vi "InitSnakes.vi"(8 "error in (no error)":errorcluster, 11 "SnakeGame in":refnum<class "SnakeGame.lvclass">) -> (0 "error out":errorcluster, 3 "SnakeGame out":refnum<class "SnakeGame.lvclass">)   [LabVIEW 2019, in "RT_Game.lvlib" / "SnakeGame.lvclass"]
uses:
  SnakeGame.lvclass
  C:/Users/FreshBob/Dropbox/VIs/myRIO_GameConsole/RT/RT_Game/Game/Game.lvclass
  Engine/Coordinate.ctl
  Snake/Direction.ctl
  Snake/Snake.lvclass
  Game/Game.lvclass/Game.ctl
  Snake/Snake.lvclass/Snake.ctl
  SnakeGame.lvclass/SnakeGame.ctl
  Game/Read Singleplayer.vi
  Snake/Write Position (Tiles).vi
  Snake/Write Direction.vi
  Snake/Write ScorePosition.vi
  Snake/Write Color.vi
  Snake/Write Length.vi
  Snake/Write tick_rate.vi
  Snake/Write Dead_.vi
  Engine/Engine.lvclass
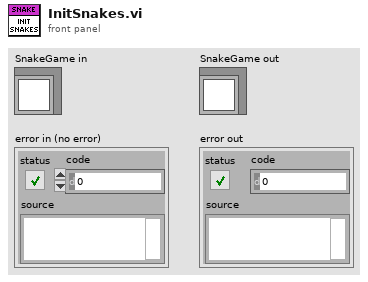
[diagram p1: front panel]
types:
  T1 = typedef "RT_Game.lvlib/Engine.lvclass/Coordinate.ctl" = cluster{"x":dbl, "y":dbl}
  T2 = typedef "RT_Game.lvlib/Snake.lvclass/Direction.ctl" = enum16{"Up", "Left", "Down", "Right"}
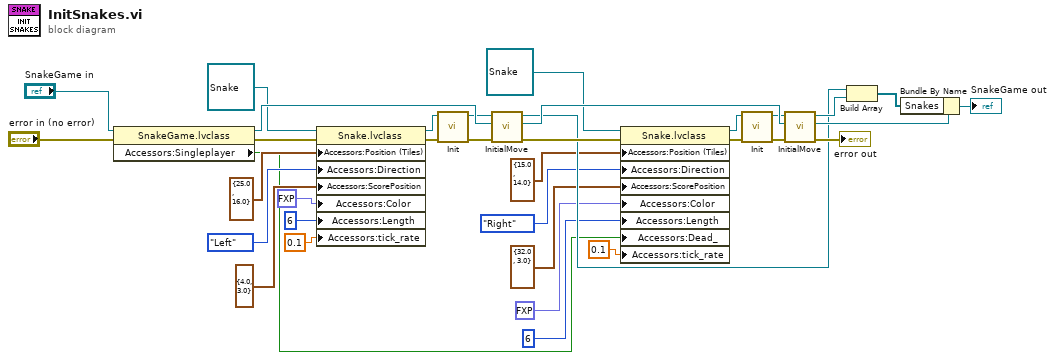
[diagram p0: block diagram]
diagram:
  n1 = property class="SnakeGame.lvclass"(reference="SnakeGame in", error in="error in (no error)") -> (reference out=w35:refnum<class "SnakeGame.lvclass">, error out=w29:errorcluster, "Accessors:Singleplayer"=w1:bool)
  n2 = property class="Snake.lvclass"(reference=refnum<class "Snake.lvclass"> refnum ("RT_Game.lvlib:Snake.lvclass"), error in=w29, "Accessors:Position (Tiles)"=T1 {"x"=25.0, "y"=16.0} ("Position (Tiles)"), "Accessors:Direction"=Direction."Left" ("Direction"), "Accessors:ScorePosition"=T1 {"x"=4.0, "y"=3.0} ("ScorePosition"), "Accessors:Color"=fxp<+,3,3> 1.0 ("Color"), "Accessors:Length"=i16 6 ("Length"), "Accessors:tick_rate"=0.1 ("tick_rate")) -> (reference out=w21:refnum<class "Snake.lvclass">, error out=w20:errorcluster)
  n3 = call-dynamic "Init.vi"("error in (no error)"=w20, "Snake in"=w21) -> ("error out"=w3:errorcluster, "Snake out"=w25:refnum<class "Snake.lvclass">)  [unwired: 8 in]
  n4 = call "InitialMove.vi"("error in (no error)"=w3, "SnakeGame in"=w35, "Snake in"=w25) -> ("error out"=w30:errorcluster, "SnakeGame out"=w33:refnum<class "SnakeGame.lvclass">, "Snake out"=w26:refnum<class "Snake.lvclass">)  [unwired: 6 in]
  n5 = property class="Snake.lvclass"(reference=refnum<class "Snake.lvclass"> refnum ("RT_Game.lvlib:Snake.lvclass"), error in=w30, "Accessors:Position (Tiles)"=T1 {"x"=15.0, "y"=14.0} ("Position (Tiles)"), "Accessors:Direction"=Direction."Right" ("Direction"), "Accessors:ScorePosition"=T1 {"x"=32.0, "y"=3.0} ("ScorePosition"), "Accessors:Color"=fxp<+,3,3> 2.0 ("Color"), "Accessors:Length"=i16 6 ("Length"), "Accessors:Dead_"=w1, "Accessors:tick_rate"=0.1 ("tick_rate")) -> (reference out=w8:refnum<class "Snake.lvclass">, error out=w9:errorcluster)
  n6 = call-dynamic "Init.vi"("error in (no error)"=w9, "Snake in"=w8) -> ("error out"=w2:errorcluster, "Snake out"=w27:refnum<class "Snake.lvclass">)  [unwired: 8 in]
  n7 = call "InitialMove.vi"("error in (no error)"=w2, "SnakeGame in"=w33, "Snake in"=w27) -> ("error out"=→"error out":errorcluster, "SnakeGame out"=w32:refnum<class "SnakeGame.lvclass">, "Snake out"=w28:refnum<class "Snake.lvclass">)  [unwired: 6 in]
  n8 = Build Array(w26, w28) -> (w6:refnum<class "Snake.lvclass">[])
  n9 = Bundle By Name(cluster=w32, "Snakes"=w6) -> (→"SnakeGame out":refnum<class "SnakeGame.lvclass">)
